vi "读取当前输入符号.vi"(8 "error in (no error)":errorcluster caption="错误输入（无错误）", 11 "计算器类输入":refnum<class "计算器类.lvclass">) -> (0 "error out":errorcluster caption="错误输出", 2 "当前输入符号":string, 3 "计算器类输出":refnum<class "计算器类.lvclass">)   [LabVIEW 2020, in "计算器类.lvclass"]
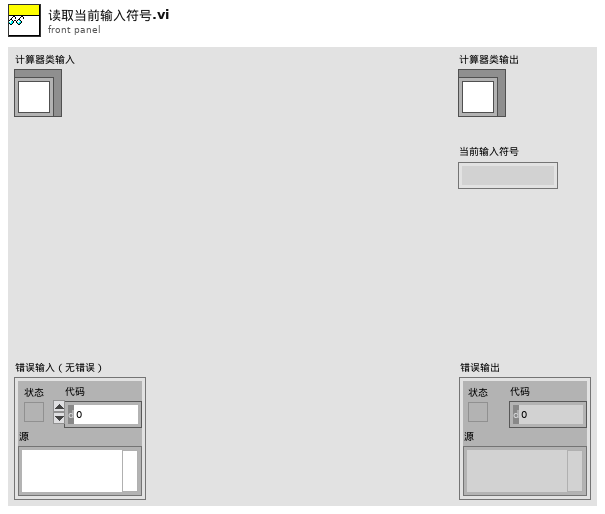
[diagram p1: front panel]
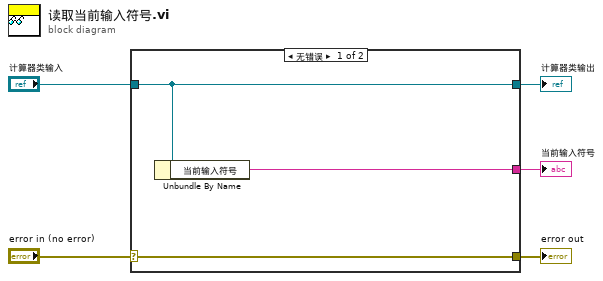
[diagram p0: block diagram]
diagram:
  n1 = case shown="无错误" "error in (no error)" {
    selector: "error in (no error)" -> [w8 w9]
    tunnel: [w8 w9] -> w4
    tunnel: [w7 w10] -> w2
    tunnel: "计算器类输入" -> [w7 w10]
    tunnel: [w6 _] -> w1
    frame No Error {
      n2 = Unbundle By Name(w7) -> ("当前输入符号"=w6:string)
    }
    frame Error {
    }
  }
  "error out" <- w4
  "计算器类输出" <- w2
  "当前输入符号" <- w1
